vi "XY Graph Get Selected Plot(s) Indices.vi"(8 "error in (no error)":errorcluster, 11 "Selected Plot Info":T1) -> (0 "error out":errorcluster, 2 "Plot(s) at Coordinates":i32[](array[numeric]), 3 "XYGraph out":T2, 4 "Plot Index in (dup)":i32)   [LabVIEW 2021, in "XY Graph Add-Ons.lvlib"]
uses:
  XY Graph Add-Ons.lvlib
  XY Graph Refnum.ctl
  XY Graph Selected Plot Info.ctl
  <vilib>/Utility/miscctls.llb/LVPoint32TypeDef.ctl
  Get Plot at Mouse Click (XY Graph)/Get Plot at Mouse Click [AAC].vi
  Graphs.lvlib
  Arrays/Arrays.lvlib
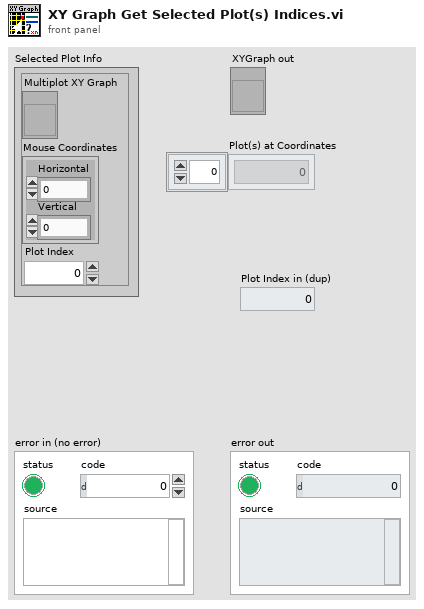
[diagram p1: front panel]
types:
  T1 = typedef "XY Graph Add-Ons.lvlib/XY Graph Selected Plot Info.ctl" = cluster{"Multiplot XY Graph":T2, "Mouse Coordinates":T3, "Plot Index":i32}
  T2 = typedef "XY Graph Add-Ons.lvlib/XY Graph Refnum.ctl" = refnum<vi>
  T3 = typedef "LVPoint32TypeDef.ctl" = cluster{"Horizontal":i32, "Vertical":i32}
  T4 = typedef "Graphs.lvlib/Graph Legend Special Coordinates.ctl" = enum16{"Last Plot", "Selected Plots", "All Plots"}
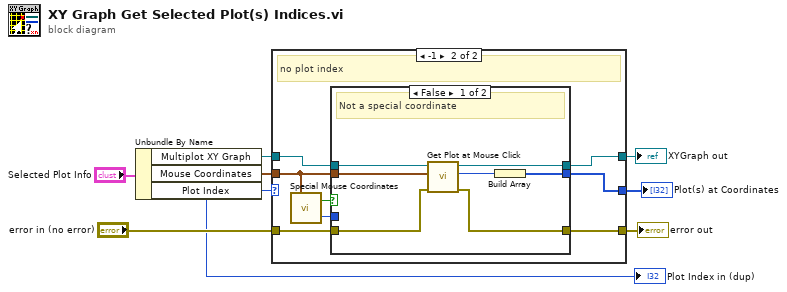
[diagram p0: block diagram]
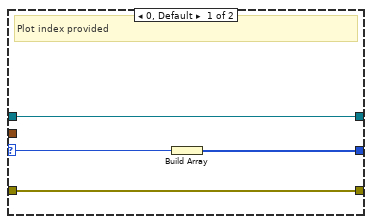
[diagram p2: hidden frame]
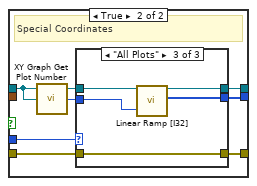
[diagram p3: hidden frame]
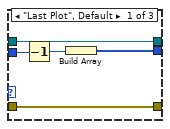
[diagram p4: hidden frame]
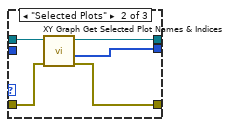
[diagram p5: hidden frame]
diagram:
  n1 = Unbundle By Name("Selected Plot Info") -> ("Multiplot XY Graph"=w4:T2, "Mouse Coordinates"=w3:T3, "Plot Index"=w1:i32)
  "Plot Index in (dup)" <- w1
  n2 = case shown="-1" w1 {
    selector: w1 -> [w10 _]
    tunnel: w4 -> [w12 w20]
    tunnel: w3 -> [_ w15]
    tunnel: "error in (no error)" -> [w11 w19]
    tunnel: [w12 w18] -> w8
    tunnel: [w11 w17] -> w7
    tunnel: [w9 w16] -> w2
    frame 0, Default {
      # "Plot index provided"
      n3 = Build Array(w10) -> (w9:i32[])
    }
    frame -1 {
      # "no plot index"
      n4 = call "Special Mouse Coordinates.vi"("Mouse Click Coordinates"=w15) -> ("Special Case (Last, Selected, All)"=w14:bool, "Special Coordinates Case"=w13:T4)
      n5 = case shown="False" w14 {
        tunnel: w20 -> [w27 w33]
        tunnel: w19 -> [w26 w30]
        tunnel: [w25 w32] -> w18
        tunnel: [w24 w29] -> w17
        tunnel: [w21 w31] -> w16
        tunnel: w15 -> [w22 _]
        tunnel: w13 -> [_ w34]
        frame False {
          # "Not a special coordinate"
          n6 = call-poly "Get Plot at Mouse Click.vi"("error in (no error)"=w26, "Mouse Click Coordinates"=w22, "XYGraph Ref"=w27) -> ("error out"=w24:errorcluster, "Plot at Coordinates"=w23:i32, "XYGraph Ref"=w25:T2)  [unwired: 2 in, 4 out]
          n7 = Build Array(w23) -> (w21:i32[])
        }
        frame True {
          # "Special Coordinates"
          n8 = call "XY Graph Get Plot Number.vi"("XYGraph"=w33) -> ("# Plots"=w28:i32)  [unwired: 8 in]
          n9 = case shown="\"All Plots\"" w34 {
            tunnel: w33 -> [w39 w44 w46]
            tunnel: [w39 w41 w46] -> w32
            tunnel: [w37 w40 w47] -> w31
            tunnel: w30 -> [w35 w43 w45]
            tunnel: [w35 w42 w45] -> w29
            tunnel: w28 -> [w36 _ w48]
            frame "Last Plot", Default {
              n10 = Decrement(x=w36) -> (x-1=w38:i32)
              n11 = Build Array(w38) -> (w37:i32[])
            }
            frame "Selected Plots" {
              n12 = call "XY Graph Get Selected Plot Names & Indices.vi"("error in (no error)"=w43, "XYGraph in"=w44) -> ("error out"=w42:errorcluster, "Selected Plots"=w40:i32[], "XYGraph out"=w41:T2)  [unwired: 5 in, 2 out]
            }
            frame "All Plots" {
              n13 = call "Linear Ramp [I32].vi"("# Elements"=w48) -> ("Ramp"=w47:i32[])  [unwired: 8 in]
            }
          }
        }
      }
    }
  }
  "XYGraph out" <- w8
  "error out" <- w7
  "Plot(s) at Coordinates" <- w2
